vi "prepAI_img.vi"(2 "triggersource":tag) -> ()   [LabVIEW 2015]
uses:
  <vilib>/DAQmx/configure/trigger.llb/DAQmx Start Trigger (Digital Edge).vi
  <vilib>/DAQmx/configure/timing.llb/DAQmx Timing (Sample Clock).vi
  <vilib>/DAQmx/create/channels.llb/DAQmx Create Channel (AI-Voltage-Basic).vi
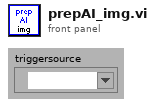
[diagram p1: front panel]
types:
  T1 = typedef "XYZStage.lvlib/XYZStage Configuration.ctl" = cluster{"VISA resource name":refnum<visa-resource-name>, "Timeout (3sec)":u32}
  T2 = cluster{"StageS":i32, "StageL":i32, "currmeas data dir":path, "image OD":u16, "contour OD":u16, "point OD":u16, "AOlines":tag[], "AIlines":tag[], "CI lines":tag[], "DO lines":tag[], "AO names":string[], "CI names":string[], "AI names":string[], "DO names":string[], "CIextensions":string[], "AIextensions":string[], "Voltage to Ygalvo":i32, "Voltage to Xgalvo":i32, "Voltage to patch":i32, "640 shutter":i32, "2P shutter":i32, "LT timestamp":u32, "Vp":i32, "Ip":i32, "camera trigger":i32, "master data dir":path, "voltage to Zpos":i32, "Vto2P":i32, "640 AO":i32, "488 AO":i32, "532 AO":i32, "640TTL":u32, "488TTL":u32, "532TTL":u32, "Device 1 sampleclock out":tag, "Device 1 Starttrigger out":tag, "Device 2 sampleclock in":tag, "Device 2 StartTrigger in ":tag, "2PODTTL":u32, "488 shutter":u32, "LCVR red":u32, "LCVR blue":u32, "Sutter Stage Config":T1, "Device 1 ext sampleclock in (100Khz)":tag}
  T3 = typedef "LVRectTypeDef.ctl" = cluster{"Left":i16, "Top":i16, "Right":i16, "Bottom":i16}
  T4 = cluster{"Xpixels":i32, "Vxminref":dbl, "Vxmaxref":dbl, "P":dbl, "Ypixels":i32, "Vyminref":dbl, "Vymaxref":dbl, "srate":sgl, "sAOxy":i32, "timeout":dbl, "type":string, "date":string, "time":string, "Colormap":u16, "Drawing Mode":u16, "Scanning Mode":u16, "square pixels":bool, "square matrix":bool, "Xpixels Img":i32, "Vx-min Img":dbl, "VX-max Img":dbl, "Ypixels Img":i32, "Vy-min Img":dbl, "Vy-max Img ":dbl, "Angle Img":dbl, "autoshutter":bool, "finite":bool, "cont":bool, "wavdet":bool, "measpoints":i32, "avpp":i32, "bufferAO":i32, "bufferAI":i32, "starttick":u32, "waveform":path, "Vx-ref":dbl, "Vy-ref":dbl, "refreshrate":dbl, "refreshbuffer":i32, "tt_cycles":i32, "motorref":refnum<k7>, "mirrorswitch":refnum<k7>, "sample mode":i32, "maxbufferAI":i32, "srateAODO":sgl, "bin":sgl, "Pel":sgl, "Angle draw":dbl, "srate Img":sgl, "ROIimg_plotbounds":T3, "auto OD":bool, "ODfilt":u16, "aAI":i32[], "aCI":i32[], "aAO":u32[], "aDO":u32[], "refwfsize":dbl, "Lifetime":bool, "Vz-Img":dbl, "Vz-ref":dbl, "Vz-reset":dbl, "AIoverride":bool, "aAS":u32[], "XYZstart":dbl[], "External 100KHz Clock?":bool}
  T5 = cluster{" AI":refnum<k21>, "E_AI":errorcluster, "header":dbl[]}
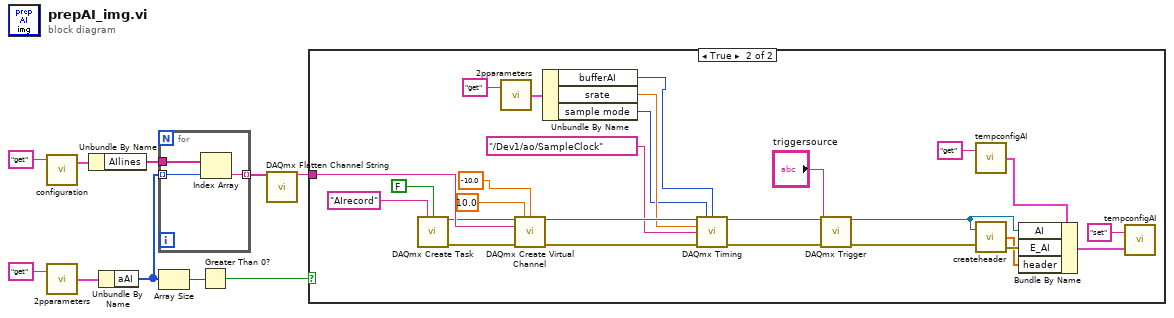
[diagram p0: block diagram]
diagram:
  n1 = call "configuration.vi"("command"="get") -> ("config out"=w7:T2)  [unwired: 2 in, 1 out]
  n2 = call "2pparameters.vi"("command"="get") -> ("params out"=w8:T4)  [unwired: 1 in]
  n3 = Unbundle By Name(w7) -> ("AIlines"=w6:tag[])
  n4 = Unbundle By Name(w8) -> ("aAI"=w4:i32[])
  n5 = for {
    tunnel: w4 -> [w13] mode=indexing
    tunnel: w6 -> [w12]
    tunnel: [w11] -> w5 mode=indexing
    n6 = Index Array(array=w12, index=w13) -> (element=w11:tag)
  }
  n7 = Array Size(array=w4) -> (size(s)=w3:i32)
  n8 = Greater Than 0?(x=w3) -> (x > 0?=w1:bool)
  n9 = call <vilib>:"DAQmx Flatten Channel String.vi"("names in"=w5) -> ("names out"=w2:string)  [unwired: 13 in, 1 out]
  n10 = case shown="True" w1 {
    tunnel: w2 -> [_ w35]
    frame False {
    }
    frame True {
      n11 = call <vilib>:"DAQmx Create Task.vi"("new task name"="AIrecord", "auto cleanup"=FALSE) -> ("task out"=w20:refnum<k21>, "error out"=w21:errorcluster)  [unwired: 12 in]
      n12 = call "2pparameters.vi"("command"="get") -> ("params out"=w37:T4)  [unwired: 1 in]
      n13 = call-poly <vilib>:"DAQmx Create Virtual Channel.vi"("task in"=w20, "maximum value"=10.0, "minimum value"=-10.0, "physical channels"=w35, "error in"=w21) -> ("task out"=w39:refnum<k21>, "error out"=w38:errorcluster)  [unwired: 9 in]
      n14 = Unbundle By Name(w37) -> ("bufferAI"=w14:i32, "srate"=w30:sgl, "sample mode"=w28:i32)
      n15 = call-poly <vilib>:"DAQmx Timing.vi"("task/channels in"=w39, "sample mode"=w28, "samples per channel"=w14, "rate"=w30, "source"=tag "/Dev1/ao/SampleClock", "error in"=w38) -> ("task out"=w25:refnum<k21>, "error out"=w17:errorcluster)  [unwired: 8 in]
      n16 = call-poly <vilib>:"DAQmx Trigger.vi"("task/channels in"=w25, "source"="triggersource", "error in"=w17) -> ("task out"=w18:refnum<k21>, "error out"=w16:errorcluster)  [unwired: 11 in]
      n17 = call "tempconfigAI.vi"("command"="get") -> ("Temp Config out"=w33:T5)  [unwired: 1 in]
      n18 = call "createheader.vi"("task in"=w18, "error in"=w16) -> ("Array"=w23:dbl[], "error out"=w24:errorcluster)  [unwired: 1 out]
      n19 = Bundle By Name(cluster=w33, "AI"=w18, "E_AI"=w24, "header"=w23) -> (w34:T5)
      n20 = call "tempconfigAI.vi"("Temp Config in"=w34, "command"="set") -> ()  [unwired: 1 out]
    }
  }
